vi "Get Thread.vi"(8 "error in (no error)":errorcluster, 11 "UIMessage in":refnum<class "UIMessage.lvclass">) -> (0 "error out":errorcluster, 2 "Thread":refnum<k7>, 3 "UIMessage out":refnum<class "UIMessage.lvclass">)   [LabVIEW 2020, in "TSnax.lvlib" / "UIMessage.lvclass"]
uses:
  UIMessage.lvclass
  UIMessage.lvclass/UIMessage.ctl
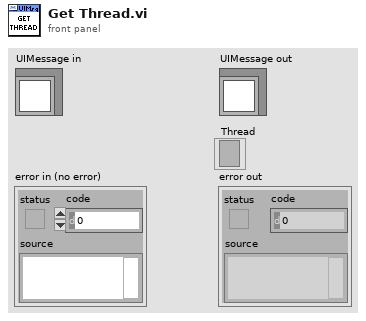
[diagram p1: front panel]
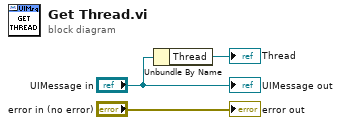
[diagram p0: block diagram]
diagram:
  n1 = Unbundle By Name("UIMessage in") -> ("Thread"=→"Thread":refnum<k7>)
  "error out" <- "error in (no error)"
  "UIMessage out" <- "UIMessage in"
